vi "RT_Main.vi"   [LabVIEW 2018]
uses:
  PublicSubVI/Ctl/_ctl_RT_FPGA_Function.ctl
  PublicSubVI/Ctl/_ctl_RT_SysLog.ctl
  <vilib>/NI_Real-Time Target Support.lvlib
types:
  T1 = cluster{"function type":enum16{"none", "init", "write", "read"}, "actionCmd":string, "callChain":string, "customErrorMsg":string, "error constant":errorcluster}
  T2 = typedef "_ctl_RT_SysLog.ctl" = enum16{"None", "Initialize", "StartupRT", "StartupFPGA", "StartupAllocator", "GetMass", "SetWfmCode", "SetLaserCtrl", "SetTurboCtrl", "SetD999Ctrl", "Reconnecting...", "Interrupt", "StopRT"}
  T3 = typedef "_ctl_RT_FPGA_Function.ctl" = enum16{"Initialisation", "Execution", "Digital In"}
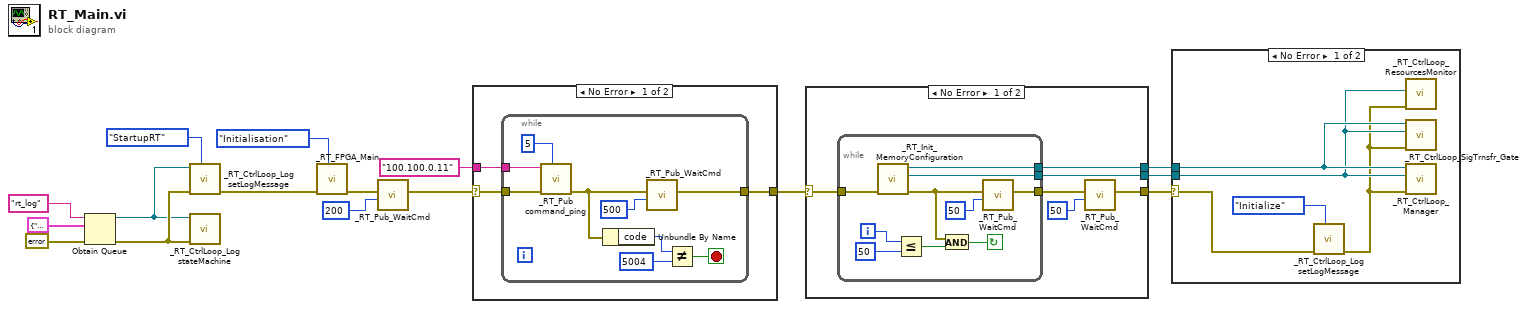
[diagram p0: block diagram]
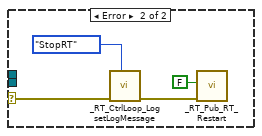
[diagram p3: hidden frame]
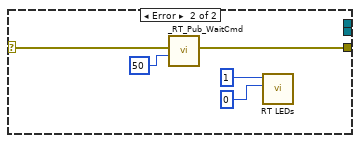
[diagram p4: hidden frame]
diagram:
  n1 = Obtain Queue(name (unnamed)="rt_log", element data type=T1 {"function type"=enum."none", "actionCmd"="", "callChain"="", "customErrorMsg"="", "error constant"={"status"=FALSE, "code"=0, "source"=""}} ("element"), error in (no error)=errorcluster {"status"=FALSE, "code"=0, "source"=""} ("Error in")) -> (queue out=w1:refnum<queue>, error out=w9:errorcluster)  [unwired: 2 in, 1 out]
  n2 = call "_RT_CtrlLoop_Log setLogMessage.vi"("system type"=_ctl_RT_SysLog."StartupRT", "error in"=w9, "RTLogQueue in"=w1) -> ("error out"=w8:errorcluster)  [unwired: 7 in, 1 out]
  n3 = call "_RT_CtrlLoop_Log stateMachine.vi"("error in (no error)"=w9, "RTLogQueue in"=w1) -> ()  [unwired: 9 in, 1 out]
  n4 = call "_RT_FPGA_Main.vi"("Function"=_ctl_RT_FPGA_Function."Initialisation", "Error in"=w8) -> ("Error out"=w6:errorcluster)  [unwired: 7 in, 2 out]
  n5 = call "_RT_Pub_WaitCmd.vi"("milliseconds to wait"=u32 200, "error in (no error)"=w6) -> ("error out"=w4:errorcluster)  [unwired: 9 in]
  n6 = case shown="No Error" w4 {
    selector: w4 -> [w18 w29]
    tunnel: [w19 w29] -> w15
    tunnel: "100.100.0.11" ("Network Identity") -> [w17 _]
    frame No Error {
      n7 = while {
        tunnel: [w23] -> w19
        tunnel: w18 -> [w26]
        tunnel: w17 -> [w20]
        stop <- w21 stop-if-true
        n8 = call "_RT_Pub command_ping.vi"("Loop Times"=5, "error in (no error)"=w26, "PCIP String"=w20) -> ("error out"=w24:errorcluster)  [unwired: 8 in]
        n9 = Unbundle By Name(w24) -> ("code"=w28:i32)
        n10 = call "_RT_Pub_WaitCmd.vi"("milliseconds to wait"=u32 500, "error in (no error)"=w24) -> ("error out"=w23:errorcluster)  [unwired: 9 in]
        n11 = Not Equal?(x=w28, y=5004 ("code")) -> (x != y?=w21:bool)
      }
    }
    frame Error {
    }
  }
  n12 = case shown="No Error" w15 {
    selector: w15 -> [w34 w47]
    tunnel: [w31 w46] -> w10
    tunnel: [w35 _] -> w16
    tunnel: [w30 _] -> w14
    frame No Error {
      n13 = while {
        tunnel: w34 -> [w45]
        tunnel: [w38] -> w32
        tunnel: [w44] -> w35
        tunnel: [w36] -> w30
        i -> [w42]
        stop <- w43 continue-if-true
        n14 = call "_RT_Init_MemoryConfiguration.vi"("error in (no error)"=w45) -> ("error out"=w39:errorcluster, "system state"=w36:refnum<data-value>, "Signal Queue"=w44:refnum<queue>)  [unwired: 7 in, 1 out]
        n15 = Less Or Equal?(x=w42, y=50) -> (x <= y?=w40:bool)
        n16 = And(x=w39, y=w40) -> (x .and. y?=w43:bool)
        n17 = call "_RT_Pub_WaitCmd.vi"("milliseconds to wait"=u32 50, "error in (no error)"=w39) -> ("error out"=w38:errorcluster)  [unwired: 9 in]
      }
      n18 = call "_RT_Pub_WaitCmd.vi"("milliseconds to wait"=u32 50, "error in (no error)"=w32) -> ("error out"=w31:errorcluster)  [unwired: 9 in]
    }
    frame Error {
      n19 = call "_RT_Pub_WaitCmd.vi"("milliseconds to wait"=u32 50, "error in (no error)"=w47) -> ("error out"=w46:errorcluster)  [unwired: 9 in]
      n20 = call <vilib>:"RT LEDs.vi"("State"=0, "LED Num"=1) -> ()  [unwired: 4 in, 2 out]
    }
  }
  n21 = case shown="No Error" w10 {
    selector: w10 -> [w53 w58]
    tunnel: w16 -> [w55 _]
    tunnel: w14 -> [w54 _]
    frame No Error {
      n22 = call "_RT_CtrlLoop_Log setLogMessage.vi"("system type"=_ctl_RT_SysLog."Initialize", "error in"=w53) -> ("error out"=w52:errorcluster)  [unwired: 8 in, 1 out]
      n23 = call "_RT_CtrlLoop_ResourcesMonitor.vi"("error in (no error)"=w52, "system state"=w54) -> ()  [unwired: 9 in, 1 out]
      n24 = call "_RT_CtrlLoop_SigTrnsfr_Gate.vi"("error in"=w52, "system state"=w54, "Signal Queue Input"=w55) -> ()  [unwired: 9 in]
      n25 = call "_RT_CtrlLoop_Manager.vi"("error in (no error)"=w52, "system state"=w54, "Signal Queue"=w55) -> ()  [unwired: 9 in]
    }
    frame Error {
      n26 = call "_RT_CtrlLoop_Log setLogMessage.vi"("system type"=_ctl_RT_SysLog."StopRT", "error in"=w58) -> ("error out"=w59:errorcluster)  [unwired: 8 in, 1 out]
      n27 = call "_RT_Pub_RT_Restart.vi"("error in (no error)"=w59, "Safe Mode?"=FALSE) -> ()  [unwired: 9 in, 1 out]
    }
  }
